vi "LvHostsEdit4cRIO_Main.vi"() -> ()   [LabVIEW 2014]
uses:
  subvi/LvHostsEdit4cRIO_Rsc_HostInfo_Typedef.ctl
  <vilib>/Utility/sysdir.llb/System Directory Type.ctl
  <vilib>/Utility/miscctls.llb/LVPointTypeDef.ctl
  subvi/LvHostsEdit4cRIO_SUB_LoginInfo_Global.vi
  subvi/LvHostsEdit4cRIO_SUB_HostInfo_Global.vi
  <vilib>/WebDAVClient/Simple Get Buffer.vi
  <vilib>/WebDAVClient/NI_WebDAV.lvlib
  <vilib>/WebDAVClient/Simple Put Buffer.vi
panel:
  in  "Btn Delete":bool
  in  "Btn Add":bool
  out "URL":string caption="target file URL:"
  out "title":string="LvHostsEdit4cRIO"
  in  "List":i32(listbox)
  # "cRIO(RTLinux)の/etc/hostsファイルをWebDAV経由で編集します。"
  # "127.0.0.1は変更できない"
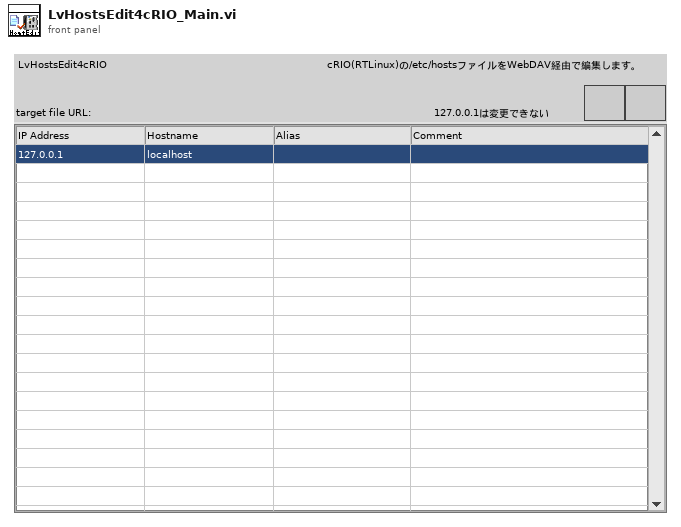
[diagram p1: front panel]
types:
  T1 = typedef "LvHostsEdit4cRIO_Rsc_HostInfo_Typedef.ctl" = cluster{"enable":bool, "IP":string, "Hostname":string, "Alias":string, "Comment":string}
  T2 = typedef "System Directory Type.ctl" = i32
  T3 = typedef "LVPointTypeDef.ctl" = cluster{"Horizontal":i16, "Vertical":i16}
  T4 = cluster{bool, "include Ctrl key?":bool, string}[]
  T5 = enum32{"invalid app kind", "Development System", "Run Time System", "Student Edition", "Embedded LabVIEW", "Evaluation", "Custom"}
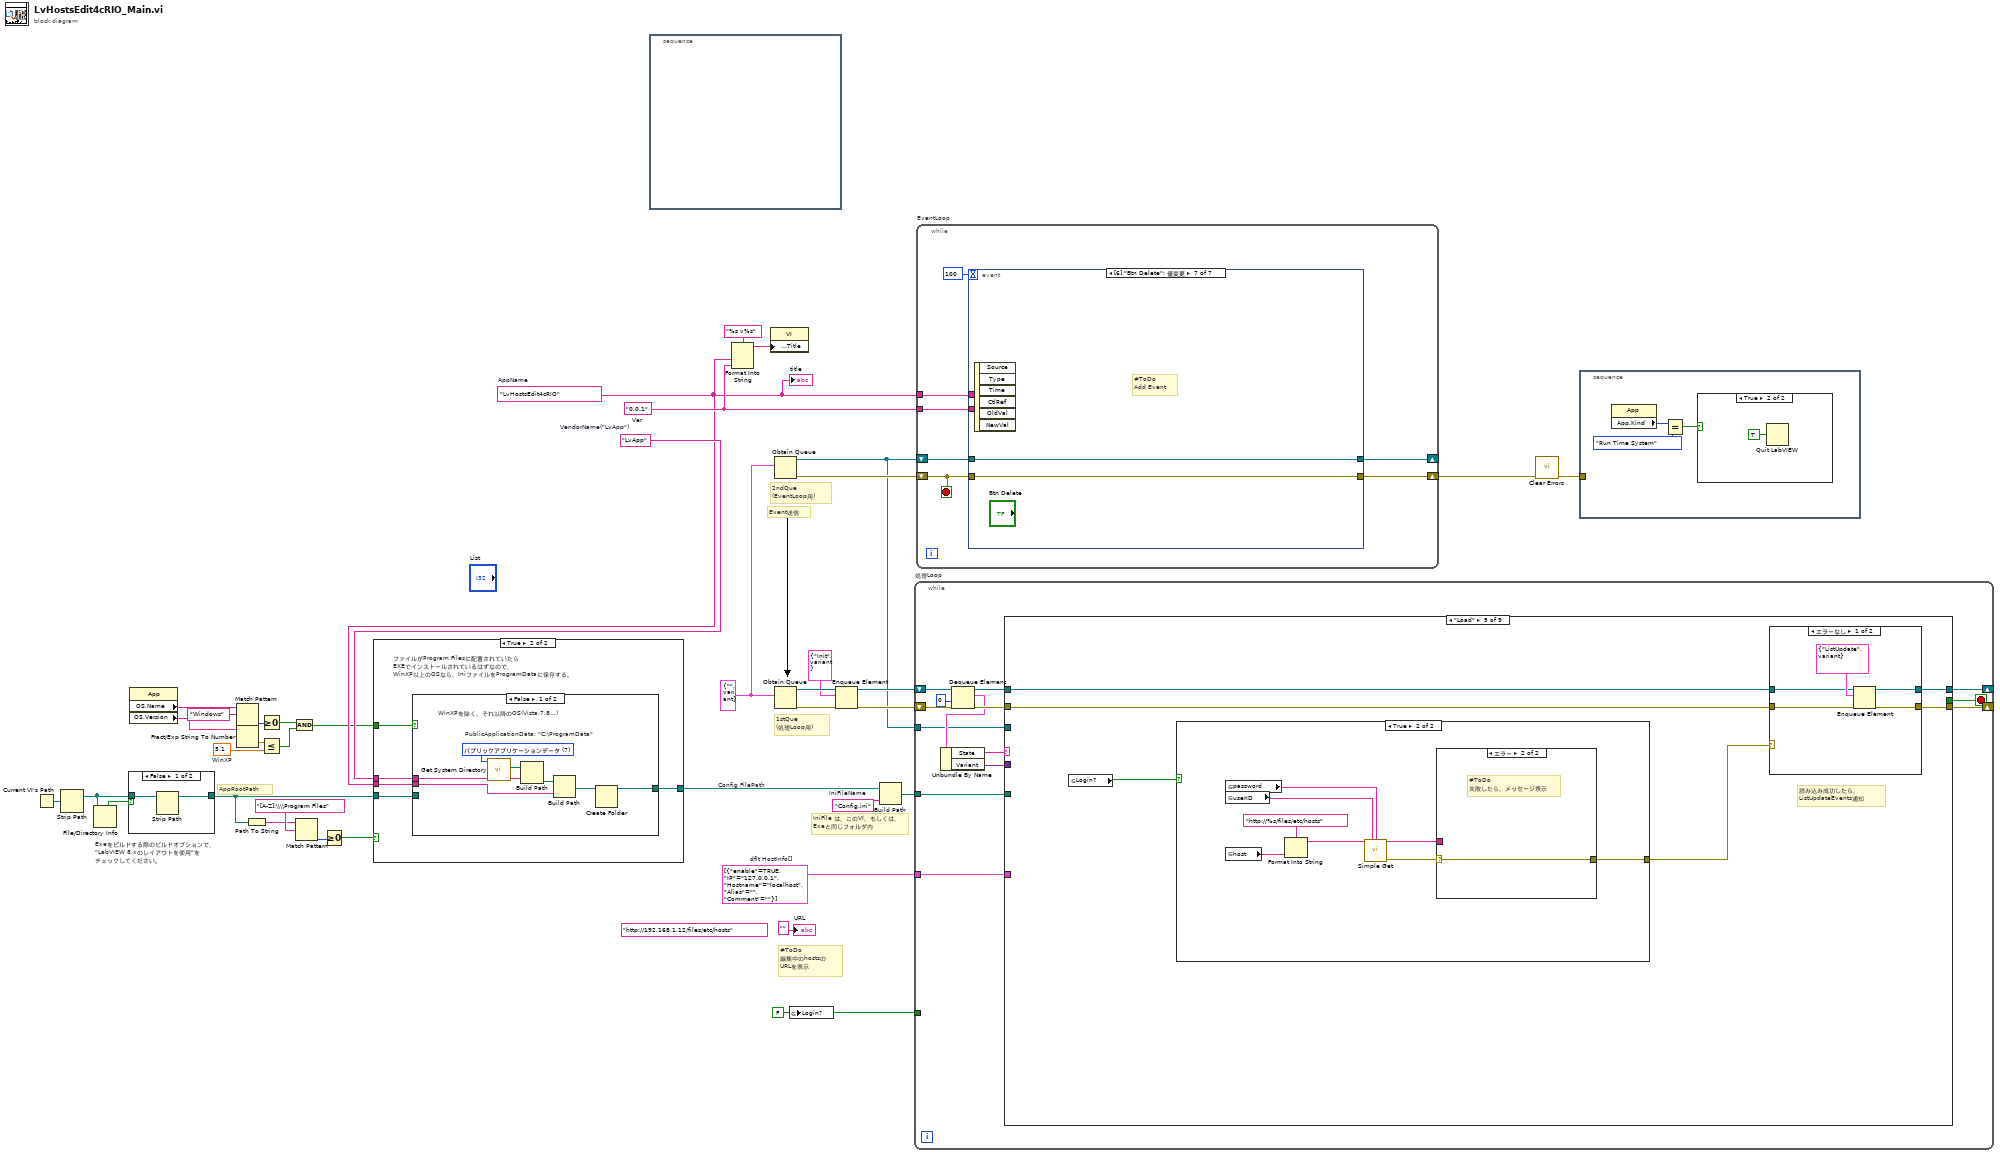
[diagram p0: block diagram]
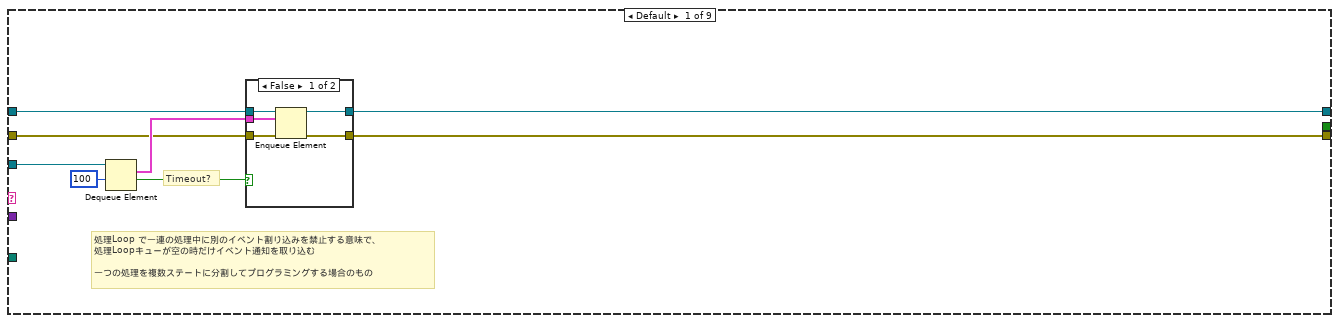
[diagram p6: hidden frame]
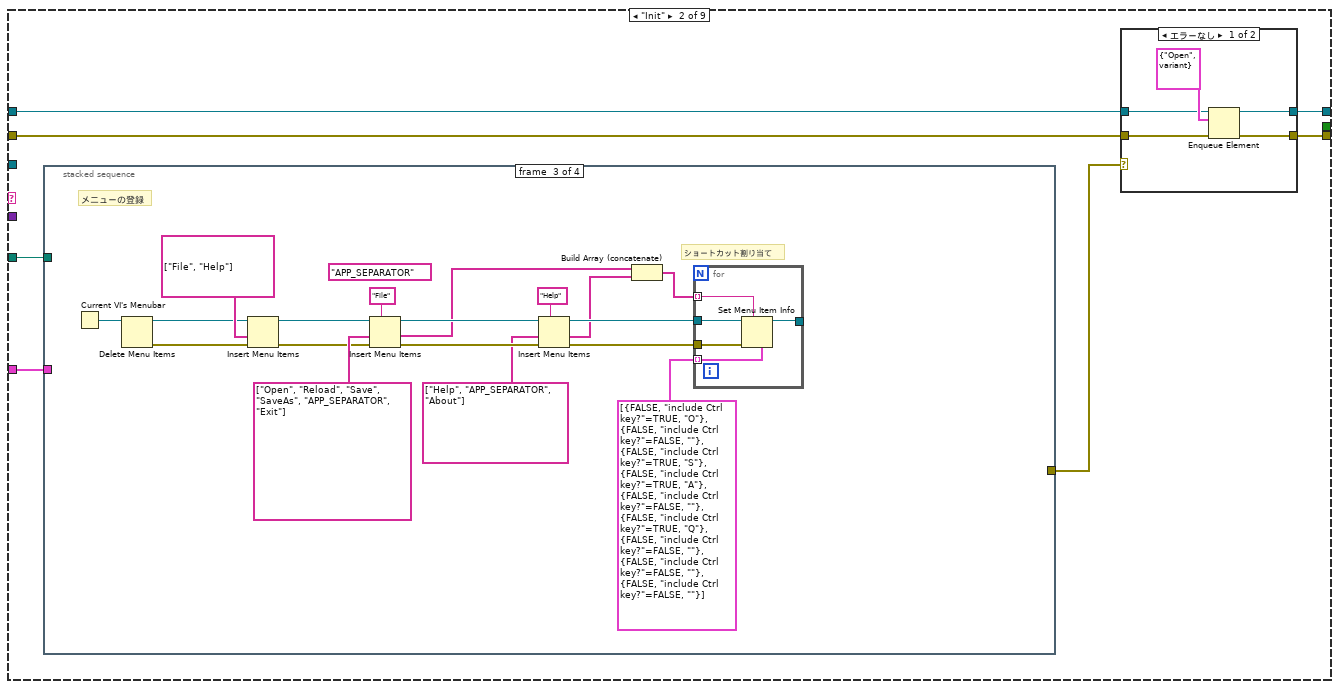
[diagram p8: hidden frame]
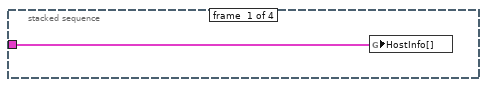
[diagram p10: hidden frame]
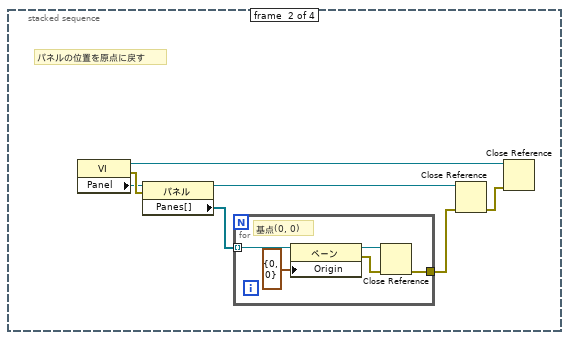
[diagram p11: hidden frame]
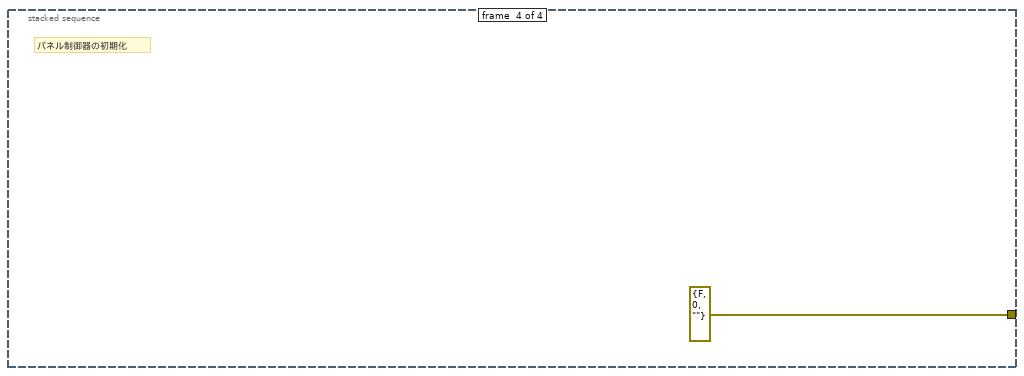
[diagram p12: hidden frame]
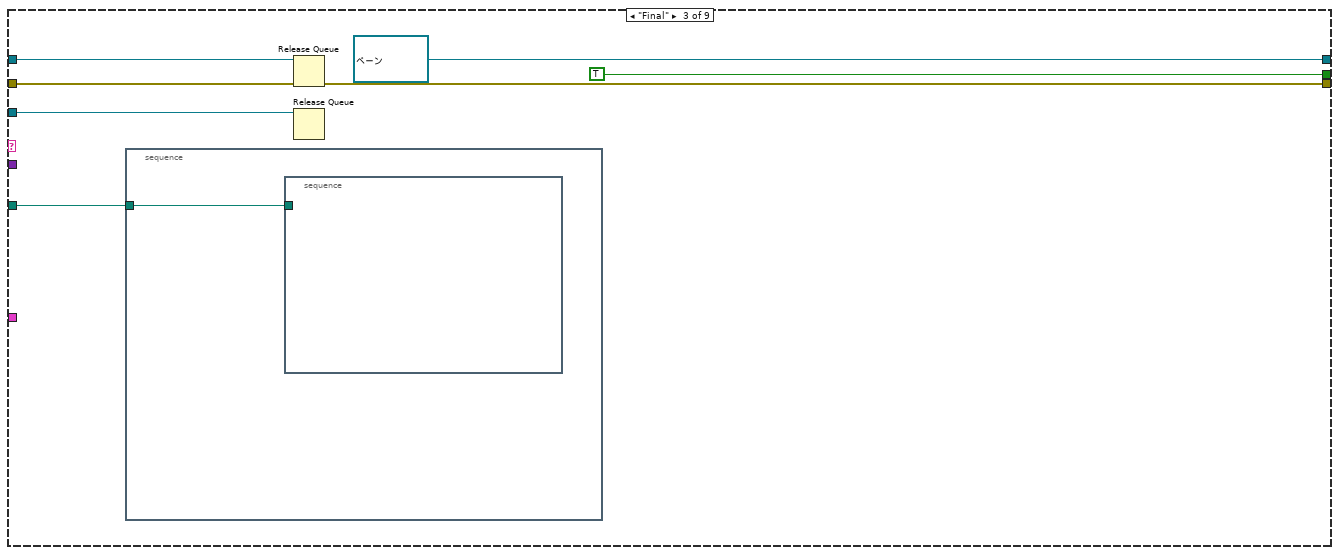
[diagram p13: hidden frame]
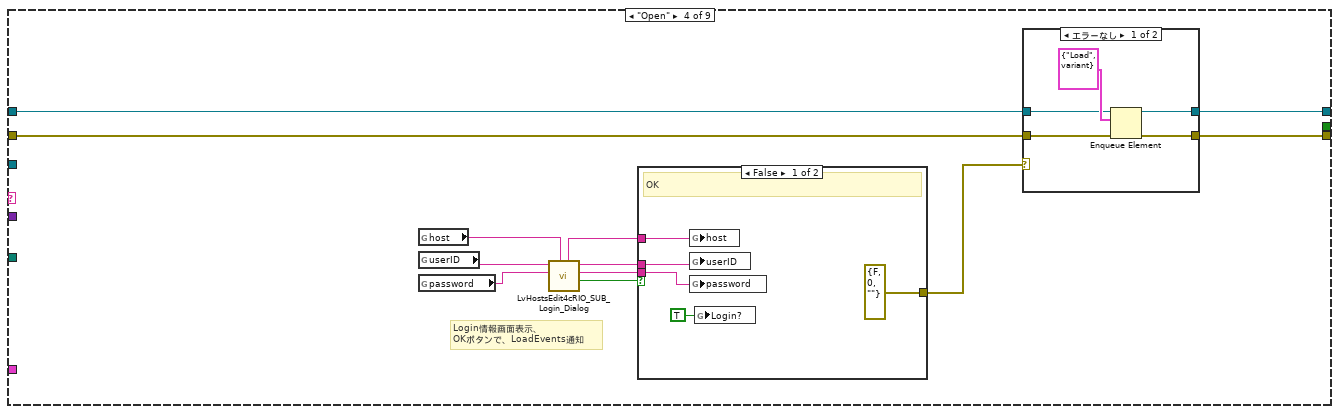
[diagram p14: hidden frame]
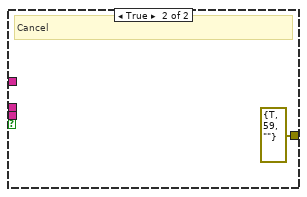
[diagram p15: hidden frame]
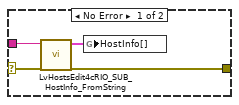
[diagram p18: hidden frame]
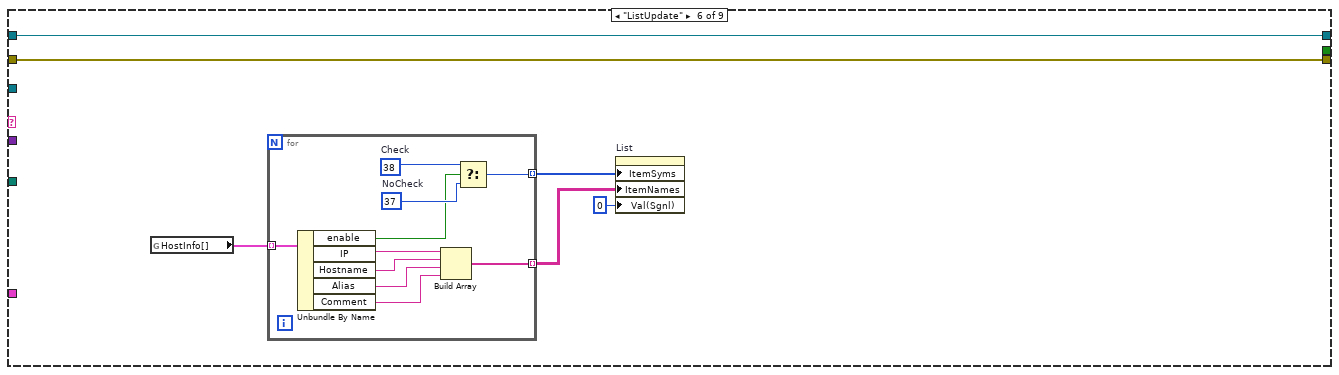
[diagram p20: hidden frame]
diagram:
  w1 = FALSE ("Login?")
  (unwired) "http://192.168.1.12/files/etc/hosts" ("URL")
  w3 = T1[] [{"enable"=TRUE, "IP"="127.0.0.1", "Hostname"="localhost", "Alias"="", "Comment"=""}]  # dflt HostInfo[]
  w14 = "LvApp"  # VendorName("LvApp")
  w19 = 5.1  # WinXP
  w24 = "Config.ini"  # IniFileName
  w27 = "0.0.1"  # Ver
  w13 = "LvHostsEdit4cRIO"  # AppName
  w38 = cluster{"State":string, "Variant":variant} {"State"="", "Variant"=variant}
  # "#ToDo\n編集中のhostsの\nURLを表示"
  # "Exeをビルドする際のビルドオプションで、\n\"LabVIEW 8.xのレイアウトを使用\"を\nチェックしてください。"
  # "Config FilePath"
  # "AppRootPath"
  # "IniFile は、このVI、もしくは、\nExeと同じフォルダ内"
  # "2ndQue\n(EventLoop用)"
  # "1stQue\n(処理Loop用)"
  # "Event送信"
  n1 = Current VI's Path() -> (path=w10:path)
  n2 = Strip Path(path=w10) -> (stripped path=w11:path)  [unwired: 1 out]
  n3 = File/Directory Info(path=w11) -> (directory=w12:bool)  [unwired: 1 in, 6 out]
  n4 = case shown="FALSE" w12 {
    tunnel: w11 -> [w40 w41]
    tunnel: [w39 w41] -> w7
    frame False {
      n5 = Strip Path(path=w40) -> (stripped path=w39:path)  [unwired: 1 out]
    }
    frame True {
    }
  }
  n6 = property class="App"() -> ("OS.Name"=w23:string, "OS.Version"=w21:string)  [unwired: 2 in, 2 out]
  n7 = Match Pattern(string=w23, regular expression="Windows" ("正規表現")) -> (offset past match=w18:i32)  [unwired: 1 in, 3 out]
  n8 = Fract/Exp String To Number(string=w21) -> (number=w20:dbl)  [unwired: 3 in, 1 out]
  n9 = Path To String(path=w7) -> (string=w6:string)
  n10 = Greater Or Equal To 0?(x=w18) -> (x >= 0?=w17:bool)
  n11 = Less Or Equal?(x=w20, y=w19) -> (x <= y?=w16:bool)
  n12 = And(x=w17, y=w16) -> (x .and. y?=w9:bool)
  n13 = Match Pattern(string=w6, regular expression="[A-Z]:\\\\Program Files" ("正規表現")) -> (offset past match=w5:i32)  [unwired: 1 in, 3 out]
  n14 = Greater Or Equal To 0?(x=w5) -> (x >= 0?=w4:bool)
  n15 = case shown="TRUE" w4 {
    tunnel: w13 -> [_ w47]
    tunnel: [w42 w45] -> w15
    tunnel: w14 -> [_ w46]
    tunnel: w9 -> [_ w44]
    tunnel: w7 -> [w42 w43]
    frame False {
      # "ファイルがProgram Filesに配置されていなかったら\n開発システムでソースから実行しているか、\nExeで適当なフォルダから実行されているので、\nIniファイルは、EXE, またはTop VI と同じ場所に保存"
    }
    frame True {
      # "ファイルがProgram Filesに配置されていたら\nEXEでインストールされているはずなので、\nWinXP以上のOSなら、IniファイルをProgramDataに保存する。"
      n16 = case shown="FALSE" w44 {
        tunnel: w47 -> [w51 _]
        tunnel: w46 -> [w49 _]
        tunnel: [w48 w55] -> w45
        tunnel: w43 -> [_ w55]
        frame False {
          w54 = T2 7 items=["ユーザホーム"=0, "ユーザデスクトップ"=1, "ユーザドキュメント"=2, "ユーザアプリケーションデータ"=3, "ユーザ設定"=4, "ユーザ一時"=5, "パブリックドキュメント"=6, "パブリックアプリケーションデータ"=7, "パブリック環境設定"=8, "パブリックキャッシュ"=13, "システムコアライブラリ"=9, "システムインストールされたライブラリ"=10, "アプリケーションファイル"=11, "ブート容量ルート"=12] ("system directory type")
          # "PublicApplicationData: \"C:\\ProgramData\""
          # "WinXPを除く、それ以降のOS(Vista,7,8,..)"
          n17 = call <vilib>:"Get System Directory.vi"("system directory type"=w54) -> ("system directory"=w53:path)  [unwired: 10 in]
          n18 = Build Path(base path=w53, name or relative path=w49) -> (appended path=w52:path)
          n19 = Build Path(base path=w52, name or relative path=w51) -> (appended path=w50:path)
          n20 = Create Folder(path (use dialog)=w50) -> (created path=w48:path)  [unwired: 2 in, 2 out]
        }
        frame True {
        }
      }
    }
  }
  n21 = stacked-sequence {
    frame #0 {
    }
  }
  n22 = Format Into String(format string="%s v%s" ("形式文字列"), w13, w27) -> (resulting string=w25:string)  [unwired: 2 in, 1 out]
  n23 = property class="VI"("Front Panel.Title"=w25) -> ()  [unwired: 2 in, 2 out]
  n24 = Obtain Queue(element data type=w38) -> (queue out=w31:refnum<queue>, error out=w37:errorcluster)  [unwired: 4 in, 1 out]
  n25 = Obtain Queue(element data type=w38) -> (queue out=w36:refnum<queue>, error out=w34:errorcluster)  [unwired: 4 in, 1 out]
  n26 = global write "LvHostsEdit4cRIO_SUB_LoginInfo_Global.vi" "Login?"(w1) -> ()
  n27 = Enqueue Element(queue=w36, element=cluster{string, "バリアント":variant} {"Init", "バリアント"=variant}, error in (no error)=w34) -> (queue out=w35:refnum<queue>, error out=w33:errorcluster)  [unwired: 1 in, 1 out]
  n28 = Build Path(base path=w15, name or relative path=w24) -> (appended path=w28:path)
  n29 = while "処理Loop" {
    shift-right: [w64] -> _
    shift-left: w35 -> [w69]
    shift-right: [w63] -> _
    shift-left: w33 -> [w66]
    tunnel: w31 -> [w59]
    tunnel: w28 -> [w57]
    tunnel: w3 -> [w56]
    tunnel: w1 -> [_]
    stop <- w58 stop-if-true
    n30 = Dequeue Element(queue=w69, timeout in ms (-1)=0 ("タイムアウト（ms）（-1）"), error in (no error)=w66) -> (queue out=w68:refnum<queue>, element=w62:cluster{"State":string, "Variant":variant}, error out=w65:errorcluster)  [unwired: 1 out]
    n31 = Unbundle By Name(w62) -> ("State"=w61:string, "Variant"=w60:variant)
    n32 = case shown="\"Load\"" w61 {
      tunnel: w68 -> [w74 w89 w141 w155 w174 w198 w213 w217 w224]
      tunnel: w59 -> [w77 _ w139 _ _ _ _ _ _]
      tunnel: w65 -> [w72 w87 w138 w154 w172 w199 w214 w218 w225]
      tunnel: [w73 w88 refnum<queue> refnum ("queue out") w152 w173 w198 w213 w217 w222] -> w64
      tunnel: [w71 w86 w137 w153 w171 w199 w214 w218 w223] -> w63
      tunnel: w60 -> [_ _ _ _ _ _ _ _ w232]
      tunnel: [_ _ TRUE _ _ _ _ _ _] -> w58
      tunnel: w57 -> [_ w91 w136 _ _ _ _ _ _]
      tunnel: w56 -> [_ w90 _ _ _ _ _ _ _]
      frame Default {
        # "Timeout?"
        # "処理Loop で一連の処理中に別のイベント割り込みを禁止する意味で、\n処理Loopキューが空の時だけイベント通知を取り込む\n\n一つの処理を複数ステートに分割してプログラミングする場合のもの"
        n33 = Dequeue Element(queue=w77, timeout in ms (-1)=100 ("タイムアウト（ms）（-1）")) -> (element=w75:cluster{"State":string, "Variant":variant}, timed out?=w70:bool)  [unwired: 1 in, 2 out]
        n34 = case shown="FALSE" w70 {
          tunnel: w75 -> [w82 _]
          tunnel: w74 -> [w81 w84]
          tunnel: [w80 w84] -> w73
          tunnel: w72 -> [w79 w83]
          tunnel: [w78 w83] -> w71
          frame False {
            n35 = Enqueue Element(queue=w81, element=w82, error in (no error)=w79) -> (queue out=w80:refnum<queue>, error out=w78:errorcluster)  [unwired: 1 in, 1 out]
          }
          frame True {
          }
        }
      }
      frame "Init" {
        n36 = stacked-sequence {
          tunnel: w91 -> [_ _ _ _]
          tunnel: w90 -> [w99 _ _ _]
          tunnel: [_ _ _ errorcluster {"status"=FALSE, "code"=0, "source"=""} ("エラー入力(エラーなし)")] -> w85
          frame #0 {
            n37 = global write "LvHostsEdit4cRIO_SUB_HostInfo_Global.vi" "HostInfo[]"(w99) -> ()
          }
          frame #1 {
            # "パネルの位置を原点に戻す"
            n38 = property class="VI"() -> (reference out=w103:refnum<vi>, error out=w106:errorcluster, "Panel"=w100:refnum<vi>)  [unwired: 2 in]
            n39 = property on="プロパティノード" class="パネル"(reference=w100, error in=w106) -> (reference out=w102:refnum<vi>, "Panes[]"=w101:refnum<vi>[])  [unwired: 1 out]
            n40 = for {
              tunnel: w101 -> [w111] mode=indexing
              tunnel: [w108] -> w104
              # "基点(0, 0)"
              n41 = property on="プロパティノード" class="ペーン"(reference=w111, "Origin"=T3 {"Horizontal"=0, "Vertical"=0} ("原点")) -> (reference out=w110:refnum<vi>, error out=w109:errorcluster)  [unwired: 1 in]
              n42 = Close Reference(reference=w110, error in (no error)=w109) -> (error out=w108:errorcluster)
            }
            n43 = Close Reference(reference=w102, error in (no error)=w104) -> (error out=w105:errorcluster)
            n44 = Close Reference(reference=w103, error in (no error)=w105) -> ()  [unwired: 1 out]
          }
          frame #2 {
            (unwired) "APP_SEPARATOR"
            # "ショートカット割り当て"
            # "メニューの登録"
            n45 = Current VI's Menubar() -> (w120:refnum<k9>)
            n46 = Delete Menu Items(9:w120) -> (0:w122:errorcluster, 3:w121:refnum<k9>)  [unwired: 3 in]
            n47 = Insert Menu Items(6:w122, 7:string[] ["File", "Help"] ("item tags"), 9:w121) -> (0:w126:errorcluster, 3:w125:refnum<k9>)  [unwired: 3 in, 1 out]
            n48 = Insert Menu Items(5:"File" ("menu tag"), 6:w126, 7:string[] ["Open", "Reload", "Save", "SaveAs", "APP_SEPARATOR", "Exit"] ("item tags"), 9:w125) -> (0:w129:errorcluster, 1:w115:string[], 3:w128:refnum<k9>)  [unwired: 2 in]
            n49 = Insert Menu Items(5:"Help" ("menu tag"), 6:w129, 7:string[] ["Help", "APP_SEPARATOR", "About"] ("item tags"), 9:w128) -> (0:w116:errorcluster, 1:w114:string[], 3:w117:refnum<k9>)  [unwired: 2 in]
            n50 = Build Array (concatenate)(w115, w114) -> (w112:string[])
            n51 = for {
              tunnel: w117 -> [w134]
              tunnel: w116 -> [w133]
              tunnel: [w132] -> _
              tunnel: T4 [{FALSE, "include Ctrl key?"=TRUE, "O"}, {FALSE, "include Ctrl key?"=FALSE, ""}, {FALSE, "include Ctrl key?"=TRUE, "S"}, {FALSE, "include Ctrl key?"=TRUE, "A"}, {FALSE, "include Ctrl key?"=FALSE, ""}, {FALSE, "include Ctrl key?"=TRUE, "Q"}, {FALSE, "include Ctrl key?"=FALSE, ""}, {FALSE, "include Ctrl key?"=FALSE, ""}, {FALSE, "include Ctrl key?"=FALSE, ""}] -> [w131] mode=indexing
              tunnel: w112 -> [w130] mode=indexing
              n52 = Set Menu Item Info(4:w131, 7:w130, 8:w133, 11:w134) -> (3:w132:refnum<k9>)  [unwired: 3 in, 1 out]
            }
          }
          frame #3 {
            # "パネル制御器の初期化"
          }
        }
        n53 = case shown="エラーなし" w85 {
          tunnel: w89 -> [w95 w97]
          tunnel: [w94 w97] -> w88
          tunnel: w87 -> [w93 w98]
          tunnel: [w92 w98] -> w86
          frame No Error {
            n54 = Enqueue Element(queue=w95, element=cluster{string, "バリアント":variant} {"Open", "バリアント"=variant}, error in (no error)=w93) -> (queue out=w94:refnum<queue>, error out=w92:errorcluster)  [unwired: 1 in, 1 out]
          }
          frame Error {
          }
        }
      }
      frame "Final" {
        n55 = stacked-sequence {
          tunnel: w136 -> [w143]
          frame #0 {
            n56 = stacked-sequence {
              tunnel: w143 -> [_]
              frame #0 {
              }
            }
          }
        }
        n57 = Release Queue(queue=w141, error in (no error)=w138) -> (error out=w137:errorcluster)  [unwired: 1 in, 2 out]
        n58 = Release Queue(queue=w139) -> ()  [unwired: 2 in, 3 out]
      }
      frame "Open" {
        # "Login情報画面表示、\nOKボタンで、LoadEvents通知"
        n59 = global read "LvHostsEdit4cRIO_SUB_LoginInfo_Global.vi" "host"() -> (w150:string)
        n60 = global read "LvHostsEdit4cRIO_SUB_LoginInfo_Global.vi" "userID"() -> (w149:string)
        n61 = global read "LvHostsEdit4cRIO_SUB_LoginInfo_Global.vi" "password"() -> (w148:string)
        n62 = call "LvHostsEdit4cRIO_SUB_Login_Dialog.vi"("host in"=w150, "password in"=w148, "userID in"=w149) -> ("Cancel?"=w147:bool, "password out"=w144:string, "userID out"=w145:string, "host out"=w146:string)  [unwired: 5 in]
        n63 = case shown="FALSE" w147 {
          tunnel: [errorcluster {"status"=FALSE, "code"=0, "source"=""} ("エラー入力(エラーなし)") errorcluster {"status"=TRUE, "code"=59, "source"=""} ("エラー入力(エラーなし)")] -> w151
          tunnel: w146 -> [w159 _]
          tunnel: w145 -> [w158 _]
          tunnel: w144 -> [w157 _]
          frame False {
            # "OK"
            n64 = global write "LvHostsEdit4cRIO_SUB_LoginInfo_Global.vi" "host"(w159) -> ()
            n65 = global write "LvHostsEdit4cRIO_SUB_LoginInfo_Global.vi" "userID"(w158) -> ()
            n66 = global write "LvHostsEdit4cRIO_SUB_LoginInfo_Global.vi" "password"(w157) -> ()
            n67 = global write "LvHostsEdit4cRIO_SUB_LoginInfo_Global.vi" "Login?"(TRUE ("Login?")) -> ()
          }
          frame True {
            # "Cancel"
          }
        }
        n68 = case shown="エラーなし" w151 {
          tunnel: w155 -> [w165 w167]
          tunnel: [w164 w167] -> w152
          tunnel: w154 -> [w163 w168]
          tunnel: [w162 w168] -> w153
          frame No Error {
            n69 = Enqueue Element(queue=w165, element=cluster{string, "バリアント":variant} {"Load", "バリアント"=variant}, error in (no error)=w163) -> (queue out=w164:refnum<queue>, error out=w162:errorcluster)  [unwired: 1 in, 1 out]
          }
          frame Error {
          }
        }
      }
      frame "Load" {
        # "読み込み成功したら、\nListUpdateEvents通知"
        n70 = global read "LvHostsEdit4cRIO_SUB_LoginInfo_Global.vi" "Login?"() -> (w169:bool)
        n71 = case shown="TRUE" w169 {
          tunnel: [_ w180] -> w170
          frame False {
          }
          frame True {
            n72 = global read "LvHostsEdit4cRIO_SUB_LoginInfo_Global.vi" "password"() -> (w178:string)
            n73 = global read "LvHostsEdit4cRIO_SUB_LoginInfo_Global.vi" "userID"() -> (w179:string)
            n74 = global read "LvHostsEdit4cRIO_SUB_LoginInfo_Global.vi" "host"() -> (w176:string)
            n75 = Format Into String(format string="http://%s/files/etc/hosts", w176) -> (resulting string=w175:string)  [unwired: 2 in, 1 out]
            n76 = call-poly <vilib>:"Simple Get.vi"("remote file uri"=w175, "username"=w179, "password"=w178) -> ("data"=w182:string, "error out"=w181:errorcluster)  [unwired: 11 in]
            n77 = case shown="エラー" w181 {
              selector: w181 -> [w183 w186]
              tunnel: w182 -> [w185 _]
              tunnel: [w183 w186] -> w180
              frame No Error {
                n78 = call "LvHostsEdit4cRIO_SUB_HostInfo_FromString.vi"("hosts data"=w185) -> ("HostInfo[] out"=w184:T1[])  [unwired: 9 in, 1 out]
                n79 = global write "LvHostsEdit4cRIO_SUB_HostInfo_Global.vi" "HostInfo[]"(w184) -> ()
              }
              frame Error {
                # "#ToDo\n失敗したら、メッセージ表示"
              }
            }
          }
        }
        n80 = case shown="エラーなし" w170 {
          tunnel: w174 -> [w190 w192]
          tunnel: [w189 w192] -> w173
          tunnel: w172 -> [w188 w193]
          tunnel: [w187 w193] -> w171
          frame No Error {
            n81 = Enqueue Element(queue=w190, element=cluster{string, "バリアント":variant} {"ListUpdate", "バリアント"=variant}, error in (no error)=w188) -> (queue out=w189:refnum<queue>, error out=w187:errorcluster)  [unwired: 1 in, 1 out]
          }
          frame Error {
          }
        }
      }
      frame "ListUpdate" {
        n82 = global read "LvHostsEdit4cRIO_SUB_HostInfo_Global.vi" "HostInfo[]"() -> (w197:T1[])
        n83 = for {
          tunnel: w197 -> [w209] mode=indexing
          tunnel: [w205] -> w196 mode=indexing
          tunnel: [w200] -> w195 mode=indexing
          w208 = 38  # Check
          w207 = 37  # NoCheck
          n84 = Unbundle By Name(w209) -> ("enable"=w206:bool, "IP"=w204:string, "Hostname"=w203:string, "Alias"=w202:string, "Comment"=w201:string)
          n85 = Build Array(w204, w203, w202, w201) -> (w200:string[])
          n86 = Select(t=w208, s=w206, f=w207) -> (s? t:f=w205:i32)
        }
        n87 = property on="List" class="MCListbox （指定）"("ItemSyms"=w196, "ItemNames"=w195, "Val(Sgnl)"=0 ("値（信号）")) -> ()  [unwired: 2 in, 2 out]
      }
      frame "Save" {
        # "#ToDO\n\nSaveする"
        # "#ToDO\n\nSaveした結果、OK, NGをMsg表示する"
        n88 = global read "LvHostsEdit4cRIO_SUB_HostInfo_Global.vi" "HostInfo[]"() -> (w210:T1[])
        n89 = call "LvHostsEdit4cRIO_SUB_HostInfo_FromString.vi"("HostInfo[]"=w210) -> ("hosts data out"=w211:string)  [unwired: 9 in, 1 out]
        n90 = disable-structure shown="無効" {
          disable-tunnel: w211 -> [w215 _]
          frame Disabled {
            n91 = call-poly <vilib>:"Simple Put.vi"("data"=w215) -> ()  [unwired: 14 in, 1 out]
          }
          frame Enabled {
          }
        }
        n92 = One Button Dialog(message="Save" ("メッセージ")) -> ()  [unwired: 1 in, 1 out]
      }
      frame "SaveAs" {
        n93 = disable-structure shown="無効" {
          frame Disabled {
            # "ファイルに保存する"
            n94 = global read "LvHostsEdit4cRIO_SUB_HostInfo_Global.vi" "HostInfo[]"() -> (w220:T1[])
            n95 = call "ファイルダイアログ"() -> ()  [unwired: 12 in, 4 out]
            n96 = call "LvHostsEdit4cRIO_SUB_HostInfo_FromString.vi"("HostInfo[]"=w220) -> ("hosts data out"=w219:string)  [unwired: 9 in, 1 out]
            n97 = Write to Text File(text=w219) -> ()  [unwired: 3 in, 3 out]
          }
          frame Enabled {
          }
        }
        n98 = One Button Dialog(message="SaveAs" ("メッセージ")) -> ()  [unwired: 1 in, 1 out]
      }
      frame "EditPanel" {
        w231 = 0  # List.SelectedLine#
        # "EditPanel"
        n99 = Variant To Data(type=w231, Variant=w232) -> (data=w227:i32)  [unwired: 1 in, 1 out]
        n100 = global read "LvHostsEdit4cRIO_SUB_HostInfo_Global.vi" "HostInfo[]"() -> (w226:T1[])
        n101 = Index Array(array=w226, index=w227) -> (element=w230:T1)
        n102 = call "LvHostsEdit4cRIO_SUB_HostEdit_Dialog.vi"("HostInfo"=w230) -> ("Cancel?"=w229:bool, "HostInfo out"=w228:T1)  [unwired: 9 in]
        n103 = case shown="FALSE" w229 {
          tunnel: w228 -> [w244 _]
          tunnel: w227 -> [w242 _]
          tunnel: w226 -> [w243 _]
          tunnel: [errorcluster {"status"=FALSE, "code"=0, "source"=""} ("エラー入力(エラーなし)") errorcluster {"status"=TRUE, "code"=0, "source"=""} ("エラー入力(エラーなし)")] -> w221
          frame False {
            n104 = in-place {
              in-place-border: w244 -> [w245]
              n105 = in-place-array #1(w243, w242) -> ()  [unwired: 1 out]
              n106 = in-place-array #1(w245) -> (w241:T1[])  [unwired: 1 out]
            }
            n107 = global write "LvHostsEdit4cRIO_SUB_HostInfo_Global.vi" "HostInfo[]"(w241) -> ()
          }
          frame True {
            # "Cancel"
          }
        }
        n108 = case shown="エラーなし" w221 {
          tunnel: w224 -> [w236 w238]
          tunnel: [w235 w238] -> w222
          tunnel: w225 -> [w234 w239]
          tunnel: [w233 w239] -> w223
          frame No Error {
            n109 = Enqueue Element(queue=w236, element=cluster{string, "バリアント":variant} {"ListUpdate", "バリアント"=variant}, error in (no error)=w234) -> (queue out=w235:refnum<queue>, error out=w233:errorcluster)  [unwired: 1 in, 1 out]
          }
          frame Error {
          }
        }
      }
    }
  }
  n110 = while "EventLoop" {
    shift-right: [w247] -> _
    shift-left: w31 -> [w252]
    shift-right: [w251] -> w30
    shift-left: w37 -> [w250]
    tunnel: w13 -> [w249]
    tunnel: w27 -> [w248]
    stop <- w250 stop-if-true
    n111 = event shown="[6] \"Btn Delete\": 値変更" {
      selector: _ -> [_ _ _ _ _ _ _]
      dyn-events: _ -> [_ _ _ _ _ _ _]
      timeout: 100 -> [_ _ _ _ _ _ _]
      tunnel: w252 -> [w257 w263 w269 w277 w318 w329 w330]
      tunnel: w250 -> [w256 w261 w267 w275 w317 w328 w331]
      tunnel: [w255 w260 w266 w274 w316 w328 w331] -> w251
      tunnel: w249 -> [_ _ _ w272 _ _ _]
      tunnel: w248 -> [_ _ _ w271 _ _ _]
      tunnel: [w254 w262 w268 w276 w315 w329 w330] -> w247
      event Timeout {
        # "EventLoopの終了用"
        # "Que解放をチェック\n(終了?)"
        n112 = event-data() -> ()  [unwired: 1 in, 2 out]
        n113 = Get Queue Status(queue=w257, error in (no error)=w256) -> (queue out=w254:refnum<queue>, error out=w255:errorcluster)  [unwired: 1 in, 6 out]
      }
      event Application Instance Close? {
        n114 = event-data() -> ()  [unwired: 1 in, 4 out]
        n115 = Enqueue Element(queue=w263, element=cluster{string, "バリアント":variant} {"Final", "バリアント"=variant}, error in (no error)=w261) -> (queue out=w262:refnum<queue>, error out=w260:errorcluster)  [unwired: 1 in, 1 out]
        n116 = event-data("SilentShutdown"=TRUE, "Discard?"=FALSE ("破棄?")) -> ()  [unwired: 1 in, 1 out]
      }
      event Panel Close? {
        n117 = event-data() -> ()  [unwired: 1 in, 3 out]
        n118 = Enqueue Element(queue=w269, element=cluster{string, "バリアント":variant} {"Final", "バリアント"=variant}, error in (no error)=w267) -> (queue out=w268:refnum<queue>, error out=w266:errorcluster)  [unwired: 1 in, 1 out]
        n119 = event-data("Discard?"=TRUE) -> ()  [unwired: 1 in, 1 out]
      }
      event Menu Selection (User) {
        n120 = event-data() -> ("ItemPath"=w273:string)  [unwired: 1 in, 5 out]
        n121 = case shown="\"File:SaveAs\"" w273 {
          tunnel: w277 -> [w279 w284 w289 w294 w299 w304 w310 w312]
          tunnel: [w279 w283 w288 w293 w298 w303 w310 w312] -> w276
          tunnel: w275 -> [w278 w282 w287 w292 w297 w302 w309 w311]
          tunnel: [w278 w281 w286 w291 w296 w301 w309 w311] -> w274
          tunnel: w272 -> [_ _ _ _ _ _ w308 _]
          tunnel: w271 -> [_ _ _ _ _ _ w307 _]
          frame Default {
          }
          frame "File:Open" {
            n122 = Enqueue Element(queue=w284, element=cluster{string, "バリアント":variant} {"Open", "バリアント"=variant}, error in (no error)=w282) -> (queue out=w283:refnum<queue>, error out=w281:errorcluster)  [unwired: 1 in, 1 out]
          }
          frame "File:Reload" {
            n123 = Enqueue Element(queue=w289, element=cluster{string, "バリアント":variant} {"Load", "バリアント"=variant}, error in (no error)=w287) -> (queue out=w288:refnum<queue>, error out=w286:errorcluster)  [unwired: 1 in, 1 out]
          }
          frame "File:Save" {
            n124 = Enqueue Element(queue=w294, element=cluster{string, "バリアント":variant} {"Save", "バリアント"=variant}, error in (no error)=w292) -> (queue out=w293:refnum<queue>, error out=w291:errorcluster)  [unwired: 1 in, 1 out]
          }
          frame "File:SaveAs" {
            n125 = Enqueue Element(queue=w299, element=cluster{string, "バリアント":variant} {"SaveAs", "バリアント"=variant}, error in (no error)=w297) -> (queue out=w298:refnum<queue>, error out=w296:errorcluster)  [unwired: 1 in, 1 out]
          }
          frame "File:Exit" {
            n126 = Enqueue Element(queue=w304, element=cluster{string, "バリアント":variant} {"Final", "バリアント"=variant}, error in (no error)=w302) -> (queue out=w303:refnum<queue>, error out=w301:errorcluster)  [unwired: 1 in, 1 out]
          }
          frame "Help:About" {
            n127 = Format Into String(format string="%s\n\nVersion : %s" ("メッセージ"), w308, w307) -> (resulting string=w305:string)  [unwired: 2 in, 1 out]
            n128 = One Button Dialog(message=w305) -> ()  [unwired: 1 in, 1 out]
          }
          frame "Help:Help" {
          }
        }
      }
      event "List": Double Click {
        # "#ToDo\nListをダブルクリックしたら、\n選択された行のHostInfoを編集する画面を呼び出す"
        n129 = event-data() -> ()  [unwired: 1 in, 1 out]
        n130 = local read "List"() -> (w313:i32)
        n131 = Less Than 0?(x=w313) -> (x < 0?=w314:bool)
        n132 = case shown="FALSE" w314 {
          tunnel: w318 -> [w325 w327]
          tunnel: w317 -> [w324 w326]
          tunnel: [w323 w326] -> w316
          tunnel: [w322 w327] -> w315
          tunnel: w313 -> [w319 _]
          frame False {
            n133 = Bundle By Name(cluster=cluster{string, "バリアント":variant} {"EditPanel", "バリアント"=variant}, "バリアント"=w319) -> (w321:cluster{string, "バリアント":variant})
            n134 = Enqueue Element(queue=w325, element=w321, error in (no error)=w324) -> (queue out=w322:refnum<queue>, error out=w323:errorcluster)  [unwired: 1 in, 1 out]
          }
          frame True {
            # "選択されてない"
          }
        }
      }
      event "Btn Add": Value Change {
        # "#ToDo\nAdd Event"
        n135 = event-data() -> ()  [unwired: 1 in, 6 out]
      }
      event "Btn Delete": Value Change {
        # "#ToDo\nAdd Event"
        n136 = event-data() -> ()  [unwired: 1 in, 6 out]
      }
    }
  }
  n137 = call <vilib>:"Clear Errors.vi"("error in (no error)"=w30) -> ("error out"=w29:errorcluster)  [unwired: 5 in, 1 out]
  n138 = stacked-sequence {
    tunnel: w29 -> [_]
    frame #0 {
      n139 = property class="App"() -> ("App.Kind"=w334:T5)  [unwired: 2 in, 2 out]
      n140 = Equal?(x=w334, y=T5."Run Time System" ("アプリケーション:種類")) -> (x = y?=w332:bool)
      n141 = case shown="TRUE" w332 {
        frame False {
        }
        frame True {
          n142 = Quit LabVIEW(quit? (T)=TRUE ("終了?（T）")) -> ()
        }
      }
    }
  }
  "title" <- w13
  "URL" <- ""
